vi "WPs and Obstacles 2 Levi.vi"(9 "Num WP":dbl, 10 "Waypoints":dbl[][](array[numeric]), 11 "Real/Sim":bool) -> (0 "Obstacle Lats and Longs":cluster{"Obs Lats":dbl[], "Obs Longs":dbl[]} {"Obs Longs" format="%#_8g"; "Obs Lats" format="%#_8g"}, 1 "WP Lats and Longs":cluster{"WP Lats":dbl[], "WP Longs":dbl[]} {"WP Longs" format="%#_8g"; "WP Lats" format="%#_8g"}, 3 "WP Map":T1(graph))   [LabVIEW 2014]
panel:
  out "longs":dbl[](array[numeric])
  out "lats":dbl[](array[numeric])
  in  "Obstacle Real Longs":dbl[](array[numeric])=[81.2678, 81.267312, 81.267112, 81.267332, 81.267916, 81.267137, 81.267874, 81.267301, 81.267913, 81.26772] format="%#_8g"
  in  "Obstacle Real Lats":dbl[](array[numeric])=[37.1524, 37.152256, 37.152877, 37.152903, 37.152565, 37.152792, 37.152806, 37.152779, 37.152868, 37.152484] format="%#_8g"
  in  "Obstacle Sim Longs":dbl[](array[numeric])=[81.2677, 81.26751, 81.267503, 81.267502, 81.267507, 81.2675, 81.267512, 81.267301, 81.267913, 81.26772] format="%#_8g"
  in  "Obstacle Sim Lats":dbl[](array[numeric])=[37.1523, 37.152605, 37.15261, 37.152613, 37.152608, 37.152615, 37.152603, 37.1527, 37.1528, 37.1524] format="%#_8g"
  in  "WP Sim Longs":dbl[](array[numeric])=[81.267743, 81.267312, 81.267112, 81.267332, 81.267916, 81.267137, 81.267874, 81.267301, 81.267913, 81.26772] format="%#_8g"
  in  "WP Sim Lats":dbl[](array[numeric])=[37.152345, 37.152256, 37.152877, 37.152903, 37.152565, 37.152792, 37.152806, 37.152779, 37.152868, 37.152484] format="%#_8g"
  # "Outputs:"
  # "Input:"
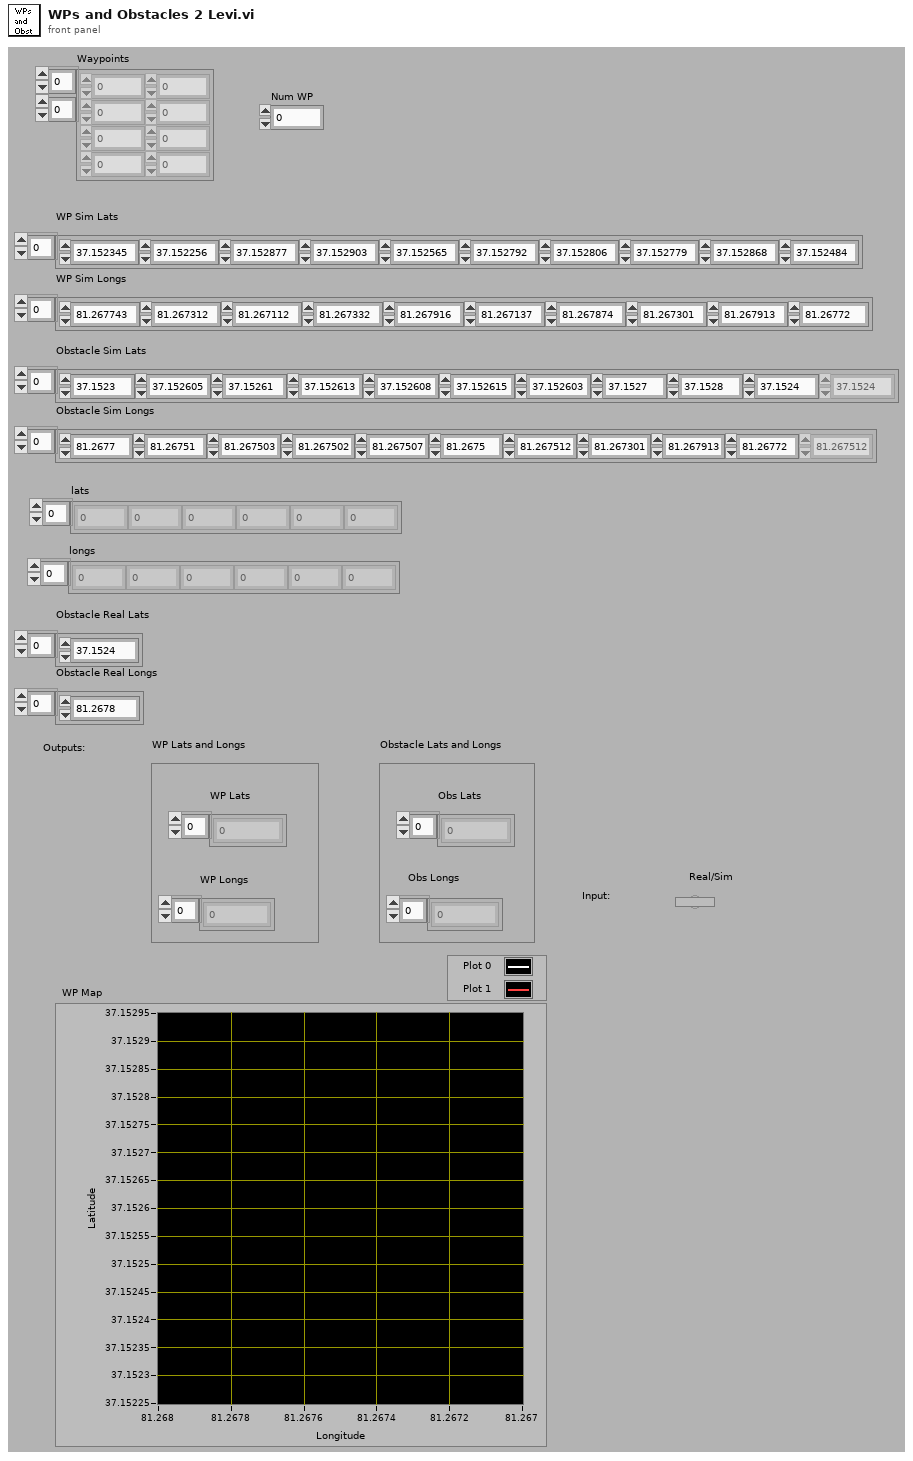
[diagram p1: front panel]
types:
  T1 = cluster{"Obstacle Longs":dbl[], "Obstacle Lats":dbl[]}[]
  T2 = cluster{"Obstacle Sim Lats":dbl[], "Obstacle Sim Longs":dbl[]}
  T3 = cluster{"WP Sim Lats":dbl[], "WP Sim Longs":dbl[]}
  T4 = cluster{"Obstacle Longs":dbl[], "Obstacle Lats":dbl[]}
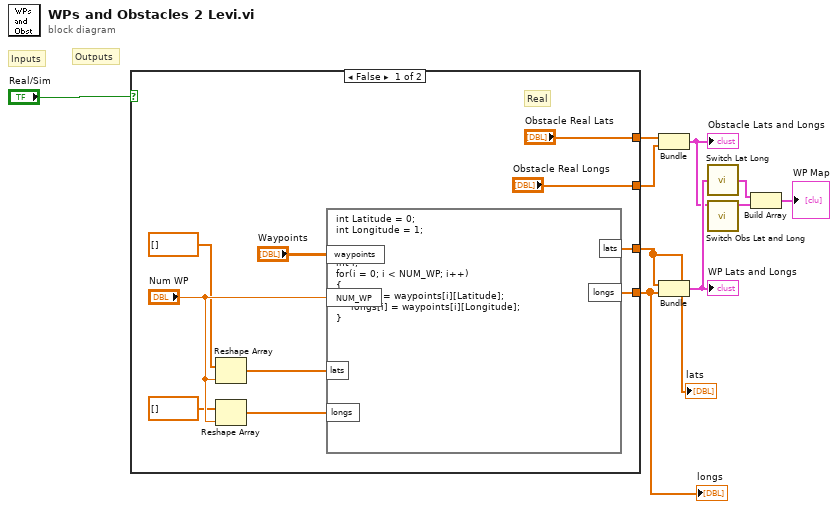
[diagram p0: block diagram]
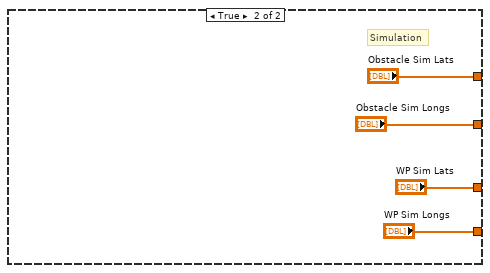
[diagram p2: hidden frame]
diagram:
  # "Inputs"
  # "Outputs"
  n1 = case shown="False" "Real/Sim" {
    tunnel: ["Obstacle Real Lats" "Obstacle Sim Lats"] -> w9
    tunnel: ["Obstacle Real Longs" "Obstacle Sim Longs"] -> w8
    tunnel: [w12 "WP Sim Lats"] -> w2
    tunnel: [w11 "WP Sim Longs"] -> w1
    frame False {
      # "Real"
      n2 = Reshape Array(dbl[] [], "Num WP") -> (w17:dbl[])
      n3 = Reshape Array(dbl[] [], "Num WP") -> (w18:dbl[])
      n4 = formula code="int Latitude = 0;\nint Longitude = 1;\n\n\nint i;\nfor(i = 0; i < NUM_WP; i++)\n{\n     lats[i] = waypoints[i][Latitude];\n     longs[i] = waypoints[i][Longitude];\n}"("waypoints"="Waypoints", "NUM_WP"="Num WP", "lats"=w17, "longs"=w18) -> ("lats"=w12:dbl[], "longs"=w11:dbl[])
    }
    frame True {
      # "Simulation"
    }
  }
  "lats" <- w2
  "longs" <- w1
  n5 = Bundle("Obstacle Sim Lats"=w9, "Obstacle Sim Longs"=w8) -> (w6:T2)  [unwired: 1 in]
  "Obstacle Lats and Longs" <- w6
  n6 = Bundle("WP Sim Lats"=w2, "WP Sim Longs"=w1) -> (w10:T3)  [unwired: 1 in]
  "WP Lats and Longs" <- w10
  n7 = call "Switch Lat Long.vi"("WP Lats and Longs for GIC"=w10) -> ("WP Lats and Longs switched"=w4:cluster{"WP Longs":dbl[], "WP Lats":dbl[]})
  n8 = call "Switch Obs Lat and Long.vi"("Obstacle Lats and Longs for GIC"=w6) -> ("Obstacle Lats and Longs switched"=w5:T4)  [unwired: 10 in]
  n9 = Build Array(w4, w5) -> (→"WP Map":T1)
